vi "NI_9252_Config.vi"(8 "error in":errorcluster, 11 "task in":refnum<k21>) -> (0 "error out":errorcluster, 3 "task out":refnum<k21>)   [LabVIEW 2022 SP3]
uses:
  <vilib>/DAQmx/create/channels.llb/DAQmx Create Channel (AI-Voltage-Basic).vi
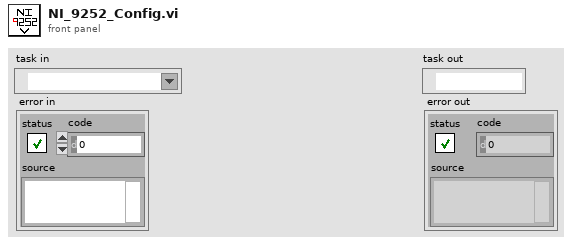
[diagram p1: front panel]
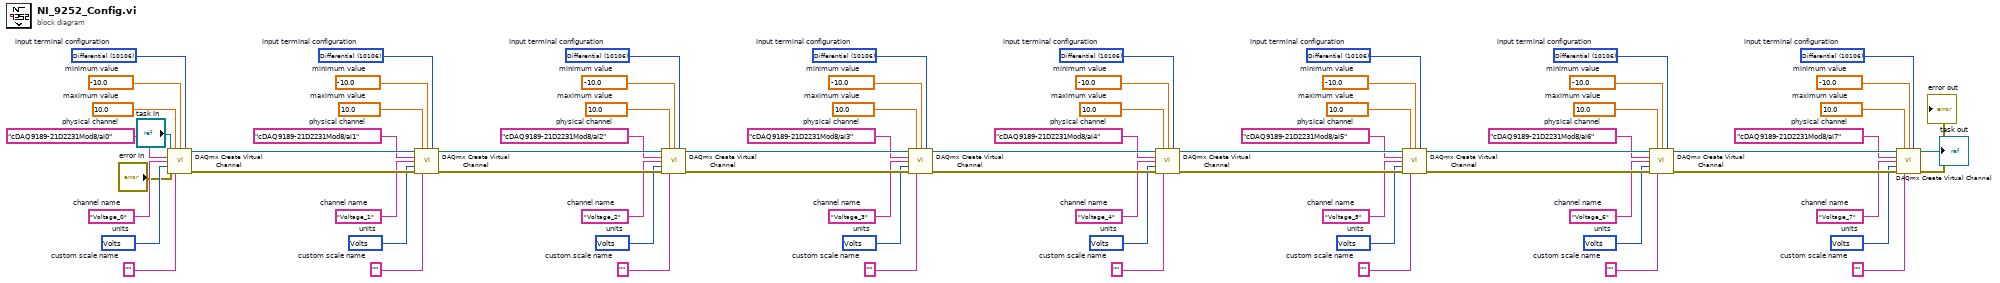
[diagram p0: block diagram]
diagram:
  w5 = 10106 items=["default"=-1, "RSE"=10083, "NRSE"=10078, "Differential"=10106, "Pseudodifferential"=12529]  # input terminal configuration
  w6 = 10348 items=["Volts"=10348, "From Custom Scale"=10065]  # units
  w7 = "Voltage_7"  # channel name
  w8 = ""  # custom scale name
  w9 = -10.0  # minimum value
  w10 = 10.0  # maximum value
  w11 = "cDAQ9189-21D2231Mod8/ai7"  # physical channel
  w13 = 10106 items=["default"=-1, "RSE"=10083, "NRSE"=10078, "Differential"=10106, "Pseudodifferential"=12529]  # input terminal configuration
  w14 = 10348 items=["Volts"=10348, "From Custom Scale"=10065]  # units
  w15 = "Voltage_6"  # channel name
  w17 = ""  # custom scale name
  w18 = -10.0  # minimum value
  w19 = 10.0  # maximum value
  w20 = "cDAQ9189-21D2231Mod8/ai6"  # physical channel
  w22 = 10106 items=["default"=-1, "RSE"=10083, "NRSE"=10078, "Differential"=10106, "Pseudodifferential"=12529]  # input terminal configuration
  w23 = 10348 items=["Volts"=10348, "From Custom Scale"=10065]  # units
  w24 = "Voltage_5"  # channel name
  w26 = ""  # custom scale name
  w27 = -10.0  # minimum value
  w28 = 10.0  # maximum value
  w29 = "cDAQ9189-21D2231Mod8/ai5"  # physical channel
  w31 = 10106 items=["default"=-1, "RSE"=10083, "NRSE"=10078, "Differential"=10106, "Pseudodifferential"=12529]  # input terminal configuration
  w32 = 10348 items=["Volts"=10348, "From Custom Scale"=10065]  # units
  w33 = "Voltage_4"  # channel name
  w35 = ""  # custom scale name
  w36 = -10.0  # minimum value
  w37 = 10.0  # maximum value
  w38 = "cDAQ9189-21D2231Mod8/ai4"  # physical channel
  w40 = 10106 items=["default"=-1, "RSE"=10083, "NRSE"=10078, "Differential"=10106, "Pseudodifferential"=12529]  # input terminal configuration
  w41 = 10348 items=["Volts"=10348, "From Custom Scale"=10065]  # units
  w42 = "Voltage_3"  # channel name
  w44 = ""  # custom scale name
  w45 = -10.0  # minimum value
  w46 = 10.0  # maximum value
  w47 = "cDAQ9189-21D2231Mod8/ai3"  # physical channel
  w49 = 10106 items=["default"=-1, "RSE"=10083, "NRSE"=10078, "Differential"=10106, "Pseudodifferential"=12529]  # input terminal configuration
  w50 = 10348 items=["Volts"=10348, "From Custom Scale"=10065]  # units
  w51 = "Voltage_2"  # channel name
  w53 = ""  # custom scale name
  w54 = -10.0  # minimum value
  w55 = 10.0  # maximum value
  w56 = "cDAQ9189-21D2231Mod8/ai2"  # physical channel
  w58 = 10106 items=["default"=-1, "RSE"=10083, "NRSE"=10078, "Differential"=10106, "Pseudodifferential"=12529]  # input terminal configuration
  w59 = 10348 items=["Volts"=10348, "From Custom Scale"=10065]  # units
  w60 = "Voltage_1"  # channel name
  w62 = ""  # custom scale name
  w63 = -10.0  # minimum value
  w64 = 10.0  # maximum value
  w65 = "cDAQ9189-21D2231Mod8/ai1"  # physical channel
  w67 = 10106 items=["default"=-1, "RSE"=10083, "NRSE"=10078, "Differential"=10106, "Pseudodifferential"=12529]  # input terminal configuration
  w68 = 10348 items=["Volts"=10348, "From Custom Scale"=10065]  # units
  w69 = "Voltage_0"  # channel name
  w71 = ""  # custom scale name
  w72 = -10.0  # minimum value
  w73 = 10.0  # maximum value
  w74 = "cDAQ9189-21D2231Mod8/ai0"  # physical channel
  n1 = call-poly <vilib>:"DAQmx Create Virtual Channel.vi"("task in"="task in", "maximum value"=w73, "minimum value"=w72, "input terminal configuration"=w67, "physical channels"=w74, "name to assign"=w69, "units"=w68, "error in"="error in", "custom scale name"=w71) -> ("task out"=w66:refnum<k21>, "error out"=w70:errorcluster)  [unwired: 5 in]
  n2 = call-poly <vilib>:"DAQmx Create Virtual Channel.vi"("task in"=w66, "maximum value"=w64, "minimum value"=w63, "input terminal configuration"=w58, "physical channels"=w65, "name to assign"=w60, "units"=w59, "error in"=w70, "custom scale name"=w62) -> ("task out"=w57:refnum<k21>, "error out"=w61:errorcluster)  [unwired: 5 in]
  n3 = call-poly <vilib>:"DAQmx Create Virtual Channel.vi"("task in"=w57, "maximum value"=w55, "minimum value"=w54, "input terminal configuration"=w49, "physical channels"=w56, "name to assign"=w51, "units"=w50, "error in"=w61, "custom scale name"=w53) -> ("task out"=w48:refnum<k21>, "error out"=w52:errorcluster)  [unwired: 5 in]
  n4 = call-poly <vilib>:"DAQmx Create Virtual Channel.vi"("task in"=w48, "maximum value"=w46, "minimum value"=w45, "input terminal configuration"=w40, "physical channels"=w47, "name to assign"=w42, "units"=w41, "error in"=w52, "custom scale name"=w44) -> ("task out"=w39:refnum<k21>, "error out"=w43:errorcluster)  [unwired: 5 in]
  n5 = call-poly <vilib>:"DAQmx Create Virtual Channel.vi"("task in"=w39, "maximum value"=w37, "minimum value"=w36, "input terminal configuration"=w31, "physical channels"=w38, "name to assign"=w33, "units"=w32, "error in"=w43, "custom scale name"=w35) -> ("task out"=w30:refnum<k21>, "error out"=w34:errorcluster)  [unwired: 5 in]
  n6 = call-poly <vilib>:"DAQmx Create Virtual Channel.vi"("task in"=w30, "maximum value"=w28, "minimum value"=w27, "input terminal configuration"=w22, "physical channels"=w29, "name to assign"=w24, "units"=w23, "error in"=w34, "custom scale name"=w26) -> ("task out"=w21:refnum<k21>, "error out"=w25:errorcluster)  [unwired: 5 in]
  n7 = call-poly <vilib>:"DAQmx Create Virtual Channel.vi"("task in"=w21, "maximum value"=w19, "minimum value"=w18, "input terminal configuration"=w13, "physical channels"=w20, "name to assign"=w15, "units"=w14, "error in"=w25, "custom scale name"=w17) -> ("task out"=w12:refnum<k21>, "error out"=w16:errorcluster)  [unwired: 5 in]
  n8 = call-poly <vilib>:"DAQmx Create Virtual Channel.vi"("task in"=w12, "maximum value"=w10, "minimum value"=w9, "input terminal configuration"=w5, "physical channels"=w11, "name to assign"=w7, "units"=w6, "error in"=w16, "custom scale name"=w8) -> ("task out"=→"task out":refnum<k21>, "error out"=→"error out":errorcluster)  [unwired: 5 in]
